vi "Extract Control Index.vi"(11 "reference":refnum<vi>) -> (3 "index":i32)   [LabVIEW 2020]
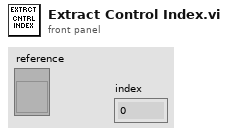
[diagram p1: front panel]
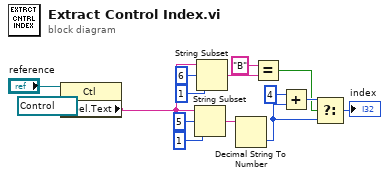
[diagram p0: block diagram]
diagram:
  (unwired) refnum<vi> refnum ("reference")
  n1 = property class="Ctl"(reference="reference") -> ("Label.Text"=w2:string)  [unwired: 1 in, 2 out]
  n2 = String Subset(string=w2, offset (0)=5, length (rest)=1 ("length (rest)")) -> (substring=w7:string)
  n3 = String Subset(string=w2, offset (0)=6, length (rest)=1 ("length (rest)")) -> (substring=w8:string)
  n4 = Decimal String To Number(string=w7) -> (number=w11:i32)  [unwired: 2 in, 1 out]
  n5 = Equal?(x="B", y=w8) -> (x = y?=w10:bool)
  n6 = Add(x=4, y=w11) -> (x+y=w13:i32)
  n7 = Select(t=w13, s=w10, f=w11) -> (s? t:f=→"index":i32)
